vi "InitThreeStack.vi"(8 "Third":refnum<class "ActionStack.lvclass">, 9 "Second":refnum<class "ActionStack.lvclass">, 10 "ActionStack in":refnum<class "ActionStack.lvclass">) -> (1 "Actions":refnum<class "ActionStack.lvclass">[](array[class]))   [LabVIEW 2024]
uses:
  ActionStack.lvclass
  ActionStack.lvclass/ActionStack.ctl
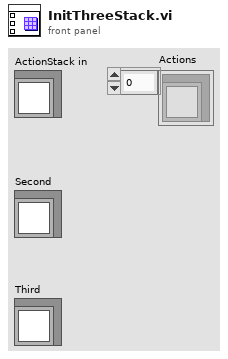
[diagram p1: front panel]
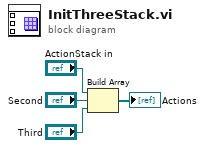
[diagram p0: block diagram]
diagram:
  n1 = Build Array("ActionStack in", "Second", "Third") -> (→"Actions":refnum<class "ActionStack.lvclass">[])
